vi "Configure Mark.vi"(7 "Mark Focus (50% of window)":dbl=50.0, 8 "error in (no error)":errorcluster, 9 "Operation (0: Create Mark)":i32(ring) items=["Create Mark", "Delete Mark", "Next Mark", "Previous Mark"], 10 "Channel (0: Channel 1)":i32(ring) items=["Channel 1", "Channel 2", "Channel 3", "Channel 4", "Math", "Bus 1", "Bus 2", "Bus 3", "Bus 4", "Reference 1", "Reference 2", "Reference 3", "Reference 4", "Column", "Digital", "RF Amplitude", "RF Frequency", "RF Phase"], 11 "VISA resource name":refnum<visa-resource-name>) -> (0 "error out":errorcluster, 3 "VISA resource name out":refnum<visa-resource-name>)   [LabVIEW 2016, in "Tektronix DPO MSO 2000 4000 Series.lvlib"]
doc: "Configures a mark on a specified waveform or all waveforms according to <B>Operation</B>. Run <B>initialize</B> VI before running this VI.\n\nUses user data to determine whether upgraded markers are available, which allows multiple markers at various locations. Supported series include the MDO 3000, the MDO 4000 and the DPO/MSO 4000B series."
uses:
  Tektronix DPO MSO 2000 4000 Series.lvlib
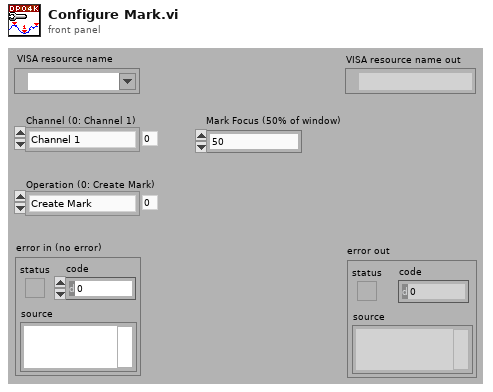
[diagram p1: front panel]
types:
  T1 = typedef "Tektronix DPO MSO 2000 4000 Series.lvlib/Extended User Data.ctl" = cluster{"DPO MSO Series Model":u16}
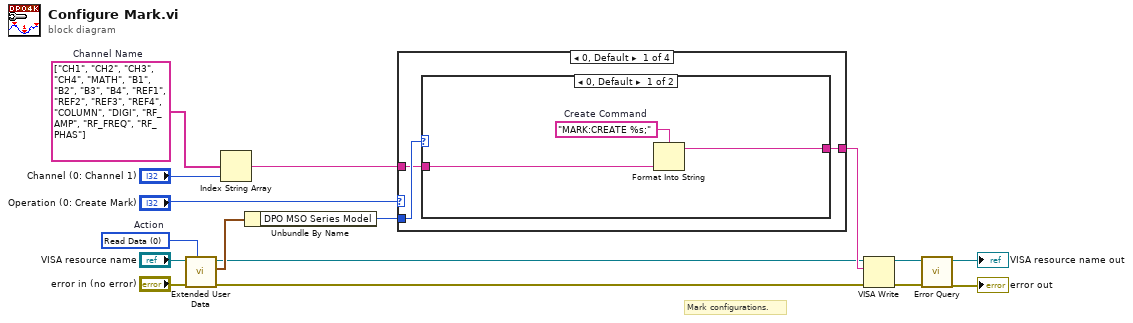
[diagram p0: block diagram]
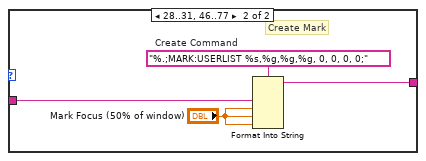
[diagram p2: hidden frame]
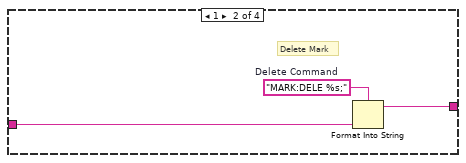
[diagram p3: hidden frame]
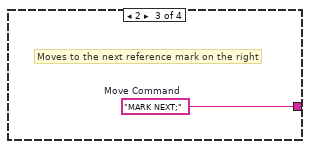
[diagram p4: hidden frame]
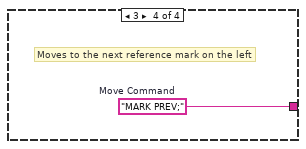
[diagram p5: hidden frame]
diagram:
  w1 = 0 items=["Read Data", "Write Data", "Clear Data", "Clear ALL Data"]  # Action
  w10 = string[] ["CH1", "CH2", "CH3", "CH4", "MATH", "B1", "B2", "B3", "B4", "REF1", "REF2", "REF3", "REF4", "COLUMN", "DIGI", "RF_AMP", "RF_FREQ", "RF_PHAS"]  # Channel Name
  # "Mark configurations."
  n1 = call "Extended User Data.vi"("Action (1: Write Data)"=w1, "error in (no error)"="error in (no error)", "VISA resource name"="VISA resource name") -> ("error out"=w2:errorcluster, "User Data Out"=w7:T1, "VISA resource name out"=w3:refnum<visa-resource-name>)  [unwired: 6 in]
  n2 = Index String Array(1:"Channel (0: Channel 1)", 2:w10) -> (0:w9:string)  [unwired: 1 in]
  n3 = Unbundle By Name(w7) -> ("DPO MSO Series Model"=w6:u16)
  n4 = case shown="0, Default" "Operation (0: Create Mark)" {
    tunnel: w9 -> [w17 w28 _ _]
    tunnel: [w19 w27 w30 w31] -> w8
    tunnel: w6 -> [w18 _ _ _]
    frame 0, Default {
      n5 = case shown="0, Default" w18 {
        tunnel: [w21 w25] -> w19
        tunnel: w17 -> [w20 w23]
        frame 0, Default {
          w22 = "MARK:CREATE %s;"  # Create Command
          n6 = Format Into String(format string=w22, w20) -> (resulting string=w21:string)  [unwired: 2 in, 1 out]
        }
        frame 28..31, 46..77 {
          w26 = "%.;MARK:USERLIST %s,%g,%g,%g, 0, 0, 0, 0;"  # Create Command
          # "Create Mark"
          n7 = Format Into String(format string=w26, w23, "Mark Focus (50% of window)", "Mark Focus (50% of window)", "Mark Focus (50% of window)") -> (resulting string=w25:string)  [unwired: 2 in, 1 out]
        }
      }
    }
    frame 1 {
      w29 = "MARK:DELE %s;"  # Delete Command
      # "Delete Mark"
      n8 = Format Into String(format string=w29, w28) -> (resulting string=w27:string)  [unwired: 2 in, 1 out]
    }
    frame 2 {
      w30 = "MARK NEXT;"  # Move Command
      # "Moves to the next reference mark on the right"
    }
    frame 3 {
      w31 = "MARK PREV;"  # Move Command
      # "Moves to the next reference mark on the left"
    }
  }
  n9 = VISA Write(VISA resource name=w3, write buffer=w8, error in (no error)=w2) -> (VISA resource name out=w16:refnum<visa-resource-name>, error out=w15:errorcluster)  [unwired: 1 out]
  n10 = call "Error Query.vi"("error in (no error)"=w15, "VISA resource name"=w16) -> ("error out"=→"error out":errorcluster, "VISA resource name out"=→"VISA resource name out":refnum<visa-resource-name>)  [unwired: 6 in, 2 out]
